vi "AlliGator Get Latest Version Number (Github).vi"(8 "Error In":errorcluster, 11 "Current Version":string) -> (0 "Error Out":errorcluster, 1 "New in this Version":string, 2 "Release Date":string, 3 "Latest Version":string, 4 "Latest Version Installer Web Address":string)   [LabVIEW 2021, in "AlliGator GUI.lvlib"]
doc: "Fetches the last released version number from the ReadTheDocs website and compares it to the current version.\n\nIf the installed version is older, offers to download and install the newest version."
uses:
  AlliGator GUI.lvlib
  <vilib>/httpClient/LabVIEWHTTPClient.lvlib
  Strings/Strings.lvlib
panel:
  # "see the AlliGator License on the block diagram (Ctrl+E or Window:Show Block Diagram)"
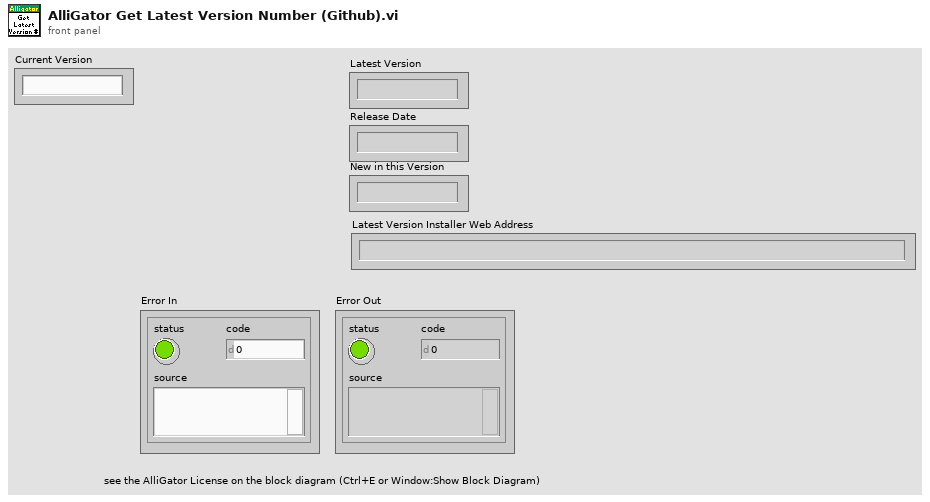
[diagram p1: front panel]
types:
  T1 = typedef "LabVIEWHTTPClient.lvlib/ClientHandle.ctl" = refnum<k1>
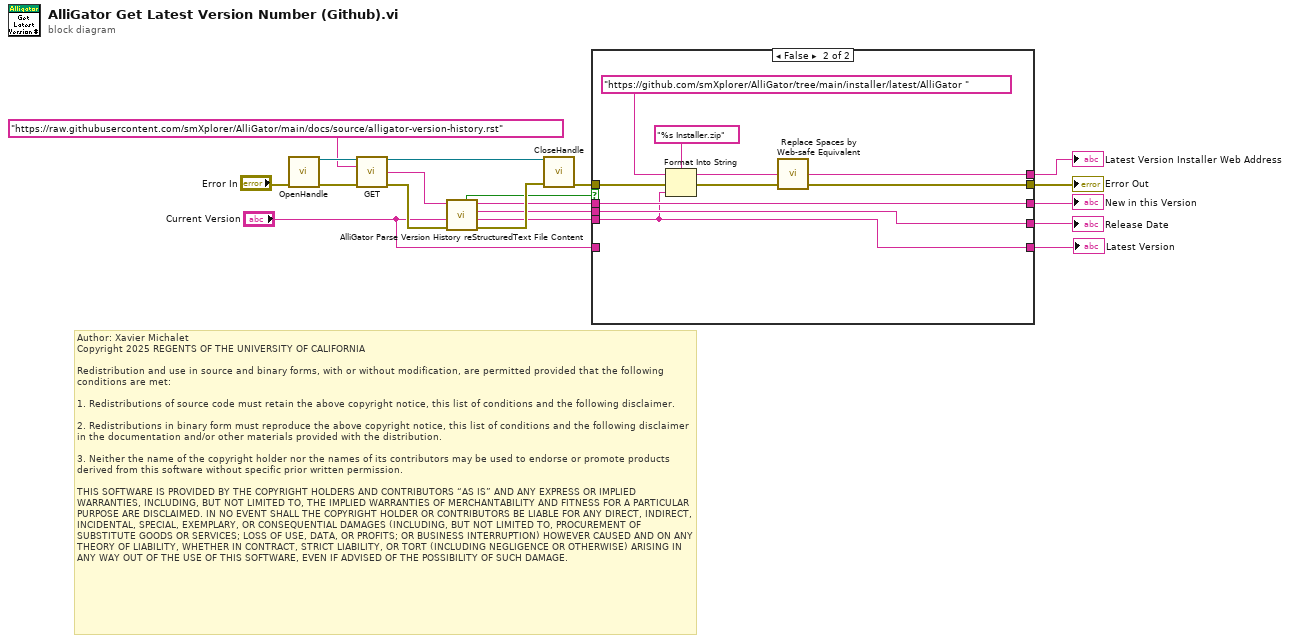
[diagram p0: block diagram]
diagram:
  # "Author: Xavier Michalet\nCopyright 2025 REGENTS OF THE UNIVERSITY OF CALIFORNIA\n\nRedistribution and use in source and binary forms, with or without modification, are permitted provided that the following conditions are met:\n\n1. Redistributions of source code must retain the above copyright notice, this list of conditions and the following disclaimer.\n\n2. Redistributions in binary form must reproduce the above copyright notice, this list of conditions and the following disclaimer in the documentation and/or other materials provided with the distribution.\n\n3. Neither the name of the copyright holder nor the names of its contributors may be used to endorse or promote products derived from this software without specific prior written permission.\n\nTHIS SOFTWARE IS PROVIDED BY THE COPYRIGHT HOLDERS AND CONTRIBUTORS “AS IS” AND ANY EXPRESS OR IMPLIED WARRANTIES, INCLUDING, BUT NOT LIMITED TO, THE IMPLIED WARRANTIES OF MERCHANTABILITY AND FITNESS FOR A PARTICULAR PURPOSE ARE DISCLAIMED. IN NO EVENT SHALL THE COPYRIGHT HOLDER OR CONTRIBUTORS BE LIABLE FOR ANY DIRECT, INDIRECT, INCIDENTAL, SPECIAL, EXEMPLARY, OR CONSEQUENTIAL DAMAGES (INCLUDING, BUT NOT LIMITED TO, PROCUREMENT OF SUBSTITUTE GOODS OR SERVICES; LOSS OF USE, DATA, OR PROFITS; OR BUSINESS INTERRUPTION) HOWEVER CAUSED AND ON ANY THEORY OF LIABILITY, WHETHER IN CONTRACT, STRICT LIABILITY, OR TORT (INCLUDING NEGLIGENCE OR OTHERWISE) ARISING IN ANY WAY OUT OF THE USE OF THIS SOFTWARE, EVEN IF ADVISED OF THE POSSIBILITY OF SUCH DAMAGE."
  n1 = call <vilib>:"OpenHandle.vi"("error in (no error)"="Error In") -> ("client handle out"=w18:T1, "error out"=w16:errorcluster)  [unwired: 13 in]
  n2 = call <vilib>:"GET.vi"("client handle"=w18, "url"="https://raw.githubusercontent.com/smXplorer/AlliGator/main/docs/source/alligator-version-history.rst", "error in (no error)"=w16) -> ("client handle out"=w17:T1, "body"=w15:string, "error out"=w14:errorcluster)  [unwired: 9 in, 1 out]
  n3 = call "AlliGator Parse Version History reStructuredText File Content.vi"("Error In"=w14, "Current Version Number"="Current Version", "Version History Page rst body"=w15) -> ("Error Out"=w13:errorcluster, "Latest Version"=w3:string, "Release Date"=w5:string, "New in this Version"=w7:string, "Version up to date"=w8:bool)  [unwired: 4 in]
  n4 = call <vilib>:"CloseHandle.vi"("client handle"=w17, "error in (no error)"=w13) -> ("error out"=w10:errorcluster)  [unwired: 13 in]
  n5 = case shown="False" w8 {
    tunnel: [_ w23] -> w11
    tunnel: w10 -> [w21 w29]
    tunnel: [w21 w28] -> w9
    tunnel: w3 -> [_ w24]
    tunnel: w7 -> [_ w26]
    tunnel: [_ w26] -> w6
    tunnel: w5 -> [_ w25]
    tunnel: [_ w25] -> w4
    tunnel: [w20 w24] -> w2
    tunnel: "Current Version" -> [w20 _]
    frame True {
    }
    frame False {
      n6 = Format Into String(format string="%s Installer.zip", initial string="https://github.com/smXplorer/AlliGator/tree/main/installer/latest/AlliGator " ("string"), error in=w29, w24) -> (resulting string=w30:string, error out=w28:errorcluster)
      n7 = call "Replace Spaces by Web-safe Equivalent.vi"("String in"=w30) -> ("String out"=w23:string)  [unwired: 8 in]
    }
  }
  "Latest Version" <- w2
  "Latest Version Installer Web Address" <- w11
  "Error Out" <- w9
  "New in this Version" <- w6
  "Release Date" <- w4
